vi "Color 2D Array To Image.vi"(8 "error in (no error)":errorcluster, 11 "Color[]":u32[][](array[numeric])) -> (0 "error out":errorcluster, 3 "Image out":refnum<class "Image.lvclass">)   [LabVIEW 2020, in "RPI.SenseHat.Display.lvlib"]
uses:
  RPI.SenseHat.Display.lvlib
  Classes/Image/Image.lvclass
  Classes/Color/Color.lvclass
  Classes/Pixel/Pixel.lvclass
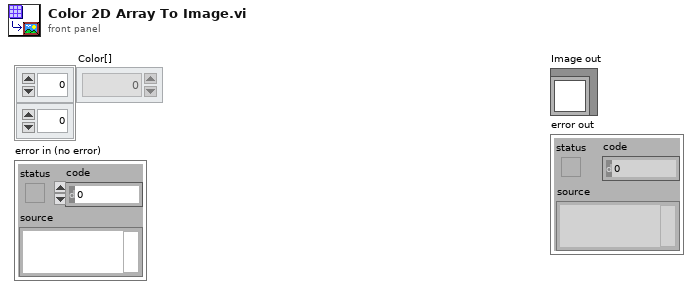
[diagram p1: front panel]
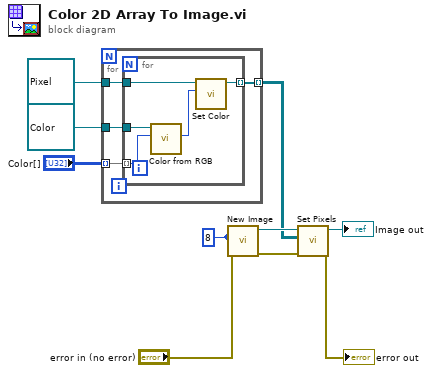
[diagram p0: block diagram]
diagram:
  w10 = 8 ("Height")
  n1 = for {
    tunnel: "Color[]" -> [w14] mode=indexing
    tunnel: refnum<class "Color.lvclass"> refnum ("RPI.SenseHat.Display.lvlib:Color") -> [w13]
    tunnel: refnum<class "Pixel.lvclass"> refnum ("RPI.SenseHat.Display.lvlib:Pixel.lvclass") -> [w12]
    tunnel: [w11] -> w6 mode=indexing
    n2 = for {
      tunnel: w14 -> [w19] mode=indexing
      tunnel: w13 -> [w18]
      tunnel: w12 -> [w17]
      tunnel: [w15] -> w11 mode=indexing
      n3 = call "Color from RGB.vi"("Color Box"=w19, "Color in"=w18) -> ("Color"=w16:u16)  [unwired: 7 in, 2 out]
      n4 = call-dynamic "Set Color.vi"("Color"=w16, "Pixel in"=w17) -> ("Pixel out"=w15:refnum<class "Pixel.lvclass">)  [unwired: 8 in, 1 out]
    }
  }
  n5 = call "New Image.vi"("error in (no error)"="error in (no error)", "Height"=w10, "Width"=w10) -> ("error out"=w3:errorcluster, "Image out"=w9:refnum<class "Image.lvclass">)  [unwired: 7 in]
  n6 = call "Set Pixels.vi"("error in (no error)"=w3, "Pixels"=w6, "Image in"=w9) -> ("error out"=→"error out":errorcluster, "Image out"=→"Image out":refnum<class "Image.lvclass">)  [unwired: 7 in]
